vi "Begin.vi"(8 "error in":errorcluster) -> (0 "error out":errorcluster)   [LabVIEW 2019]
doc: "Called before other user functions, this VI can be used to open I/O refnums, load in file data, and do general program initialization. Notice that the <B>error out</B> terminal is simply used for data flow. Wiring it to other structures or subVIs ensures that this VI runs first."
uses:
  <vilib>/Rock Robotics/WPI/DriverStation/WPI_DriverStationRobotMode2.ctl
  <vilib>/Rock Robotics/WPI/Joystick/WPI_JoystickDeviceEnum.ctl
  <vilib>/Rock Robotics/SystemInterfaces/DIO/FPGA_DIOPWMChannel.ctl
  <vilib>/Rock Robotics/WPI/SafetyOutput/WPI_SafetyOutputConfigMenu.ctl
  <vilib>/Rock Robotics/WPI/Solenoid/WPI_SolenoidChannel.ctl
  <vilib>/Rock Robotics/SystemInterfaces/i2clib/i2c_bus.ctl
  <vilib>/Rock Robotics/WPI/Solenoid/WPI_SolenoidValue.ctl
  Robot Global Data.vi
  <vilib>/Rock Robotics/WPI/RobotDrive/WPI_RobotDriveOpen2MotorWithExistingMotors.vi
  <vilib>/Rock Robotics/WPI/MotorControl/WPI_MotorControlOpen SPARK.vi
  <vilib>/Rock Robotics/WPI/Solenoid/WPI_SolenoidOpenDouble.vi
  <vilib>/Rock Robotics/WPI/Solenoid/WPI_SolenoidSetEnum.vi
  <vilib>/Rock Robotics/Network Tables/NT Write Number.vi
  <vilib>/Rock Robotics/Network Tables/NT Write Boolean Array.vi
  <vilib>/Rock Robotics/Network Tables/NT Write Numeric Array.vi
  <vilib>/Rock Robotics/WPI/Ultrasonic/WPI_SonarMB1010DigitalOpen.vi
  <vilib>/Rock Robotics/SystemInterfaces/DIO/FPGA_DIOChannel.ctl
  <vilib>/Rock Robotics/WPI/Ultrasonic/WPI_SonarMB1010DigRefNum Registry Set.vi
panel:
  in  "Blue Calibration":cluster{"R":dbl, "G":dbl, "B":dbl}={"R"=0.143, "G"=0.427, "B"=0.429}
  in  "Green Calibration":cluster{"R":dbl, "G":dbl, "B":dbl}={"R"=0.197, "G"=0.561, "B"=0.24}
  in  "Red Calibration":cluster{"R":dbl, "G":dbl, "B":dbl}={"R"=0.561, "G"=0.323, "B"=0.114}
  in  "Yellow Calibration":cluster{"R":dbl, "G":dbl, "B":dbl}={"R"=0.361, "G"=0.524, "B"=0.113}
  in  "Calibration Time (sec)":u32=4
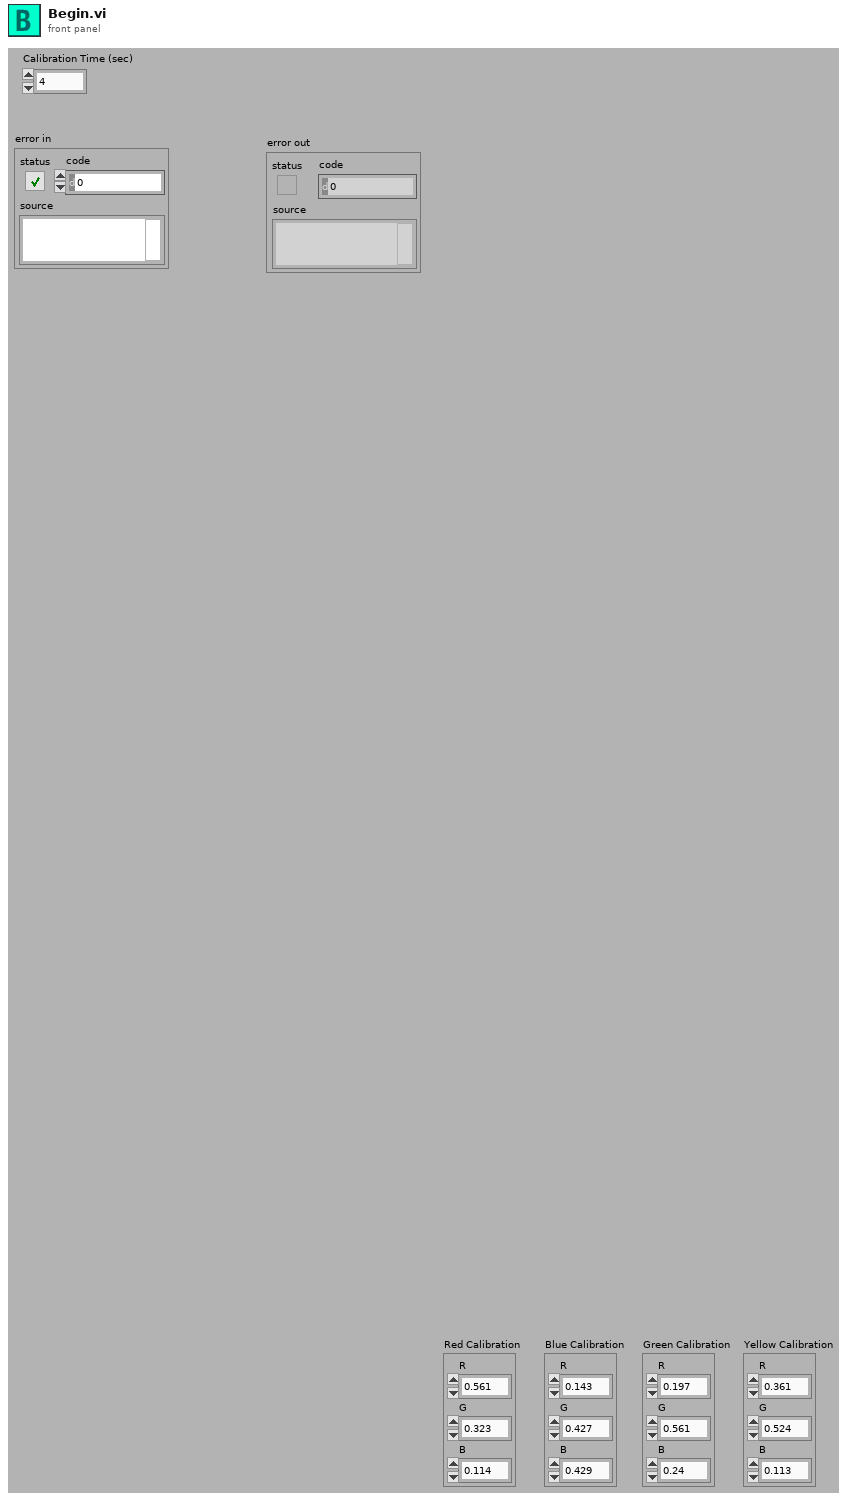
[diagram p1: front panel]
types:
  T1 = typedef "FPGA_DIOChannel.ctl" = enum8{"DIO 0", "DIO 1", "DIO 2", "DIO 3", "DIO 4", "DIO 5", "DIO 6", "DIO 7", "DIO 8", "DIO 9", "DIO MXP 0", "DIO MXP 1", "DIO MXP 2", "DIO MXP 3", "DIO MXP 4", "DIO MXP 5", "DIO MXP 6", "DIO MXP 7", "DIO MXP 8", "DIO MXP 9", "DIO MXP 10", "DIO MXP 11", "DIO MXP 12", "DIO MXP 13", "DIO MXP 14", "DIO MXP 15", "SPI Port CS1", "SPI Port CS2", "SPI Port CS3", "SPI Port MISO", "SPI Port MOSI", "Invalid"}
  T2 = typedef "WPI_SolenoidChannel.ctl" = enum8{"Solenoid 0", "Solenoid 1", "Solenoid 2", "Solenoid 3", "Solenoid 4", "Solenoid 5", "Solenoid 6", "Solenoid 7", "Invalid"}
  T3 = typedef "WPI_SolenoidValue.ctl" = enum16{"Off", "On", "Forward", "Reverse"}
  T4 = typedef "WPI_SafetyOutputConfigMenu.ctl" = enum16{"Enable", "Disable"}
  T5 = typedef "i2c_bus.ctl" = enum16{"I2C On-Board", "I2C MXP", "Invalid"}
  T6 = typedef "FPGA_DIOPWMChannel.ctl" = enum8{"PWM 0", "PWM 1", "PWM 2", "PWM 3", "PWM 4", "PWM 5", "PWM 6", "PWM 7", "PWM 8", "PWM 9", "PWM MXP 0", "PWM MXP 1", "PWM MXP 2", "PWM MXP 3", "PWM MXP 4", "PWM MXP 5", "PWM MXP 6", "PWM MXP 7", "PWM MXP 8", "PWM MXP 9", "Invalid"}
  T7 = typedef "WPI_JoystickDeviceEnum.ctl" = enum16{"USB 0", "USB 1", "USB 2", "USB 3", "USB 4", "USB 5"}
  T8 = typedef "WPI_DriverStationRobotMode2.ctl" = enum16{"Autonomous Disabled", "Autonomous Enabled", "Teleop Disabled", "Teleop Enabled", "Disconnected", "Finish", "Test Disabled", "Test Enabled", "Emergency Stopped"}
  T9 = typedef "WPI_JoystickDevRef.ctl" = cluster{"Device":T7}
  T10 = typedef "WPI_SonarMB1010DigitalDeviceRef.ctl" = cluster{"CounterDevRef":T11, "Scaling factor (s/in)":dbl}
  T11 = typedef "WPI_CounterDevRef.ctl" = cluster{"DevStatus":errorcluster, "CntIndex":T12}
  T12 = typedef "FPGA_CounterCtrSystemIndex.ctl" = enum8{"Ctr 0", "Ctr 1", "Ctr 2", "Ctr 3", "Ctr 4", "Ctr 5", "Ctr 6", "Ctr 7", "Invalid"}
  T13 = typedef "WPI_MotorControlDeviceRef.ctl" = cluster{"DeviceStatus":errorcluster, "Type":T14, "PWM":cluster{"PWM Channel":T6, "DeadBand":T15}, "CAN":cluster{"Device Number":u8, "SetOutput VI Ref":variant, "GetOutput VI Ref":variant, "Enable VI Ref":variant, "Disable VI Ref":variant, "Data":variant}, "Invert":bool, "DIO PWM":cluster{"PWM \"Enable\" Channel":T6, "DIOChannel":T1, "PWM Rate":dbl}}
  T14 = typedef "WPI_MotorControlType.ctl" = enum16{"PWM", "CAN", "DIO PWM"}
  T15 = typedef "WPI_PWMDeadband.ctl" = cluster{"Name":string, "maxPositivePwm":i32, "minPositivePwm":i32, "centerPwm":i32, "maxNegativePwm":i32, "minNegativePwm":i32, "angularRange":u16}
  T16 = typedef "WPI_RobotDriveDevRef.ctl" = cluster{"DevStatus":errorcluster, "Motors[]":T13[], "Square Inputs":bool, "Max Output":dbl}
  T17 = typedef "ADIS 16448 HW Configuration.ctl" = cluster{"SPI Clock Rate (Hz)":dbl, "IMU SPI Mode (3)":T18, "IMU Reset Pin":T1, "IMU SPI Bus":T19, "IMU Data Ready Pin":T1, "Stall Config":cluster{"Pow2BytesPerRead":u8, "StallTicks":u16, "CsToSclkTicks":u8}, "IMU Status LED Pin":T1}
  T18 = typedef "WPI_SPIMode.ctl" = enum16{"Mode 0 (Clk Idle Low,Sample on Leading)", "Mode 1 (Clk Idle Low,Sample on Trailing)", "Mode 2 (Clk Idle High,Sample on Leading)", "Mode 3 (Clk Idle High,Sample on Trailing)"}
  T19 = typedef "spi_bus.ctl" = enum16{"SPI On-Board, CS0", "SPI On-Board, CS1", "SPI On-Board, CS2", "SPI On-Board, CS3", "SPI MXP", "Invalid"}
  T20 = typedef "ADIS16448 Device Reference.ctl" = cluster{"DevStatus":errorcluster, "Hardware Config":T21, "Calibration Complete":refnum<notifier>, "Status FIFO":refnum<k33>, "Last Value Reference":refnum<data-value>, "Sychronous Process VI":T22, "Cmd FIFO":refnum<k33>, "Source":T23, "Data FIFO":refnum<k33>, "IMU Status LED Pin":T1, "Calibration Time":u32}
  T21 = typedef "ADIS16448 Hardware Configuration.ctl" = cluster{"SPI Clock Rate (Hz)":dbl, "IMU SPI Mode (3)":T18, "IMU Reset Pin":T1, "IMU SPI Bus":T19, "IMU Data Ready Pin":T1, "Stall Config":cluster{"Pow2BytesPerRead":u8, "StallTicks":u16, "CsToSclkTicks":u8}, "IMU Status LED Pin":T1}
  T22 = typedef "ADIS16448 Process.ctl" = refnum<vi>
  T23 = typedef "FPGA_CounterEncoderSourceConvertionLVSourceType.ctl" = cluster{"DevStatus":errorcluster, "AnalogTriggerMode?":bool, "DigitalMode":cluster{"DIO Channel":T24}, "AnalogTriggerMode":cluster{"AnalogTriggerIndex":T25, "OutputType":T26}}
  T24 = typedef "FPGA_DIODigitalSourceChannel.ctl" = enum8{"DIO 0", "DIO 1", "DIO 2", "DIO 3", "DIO 4", "DIO 5", "DIO 6", "DIO 7", "DIO 8", "DIO 9", "DIO MXP 0", "DIO MXP 1", "DIO MXP 2", "DIO MXP 3", "DIO MXP 4", "DIO MXP 5", "DIO MXP 6", "DIO MXP 7", "DIO MXP 8", "DIO MXP 9", "DIO MXP 10", "DIO MXP 11", "DIO MXP 12", "DIO MXP 13", "DIO MXP 14", "DIO MXP 15", "SPI Port CS1", "SPI Port CS2", "SPI Port CS3", "SPI Port MISO", "SPI Port MOSI", "Disabled"}
  T25 = typedef "FPGA_AnalogTriggerIndex.ctl" = enum8{"Trig 0", "Trig 1", "Trig 2", "Trig 3", "Trig 4", "Trig 5", "Trig 6", "Trig 7", "Invalid"}
  T26 = typedef "FPGA_AnalogTriggerOutType.ctl" = enum16{"InWindow", "TriggerState", "Rising", "Falling"}
  T27 = typedef "Color Sensor V3 DevRef.ctl" = cluster{"I2CDevRef":T28}
  T28 = typedef "WPI_I2CDevRef.ctl" = cluster{"DevStatus":errorcluster, "Device Address":u8, "Handle":i32, "I2C Bus":T5}
  T29 = typedef "WPI_SolenoidDevRef.ctl" = cluster{"DevStatus":errorcluster, "Pneumatics Control Module":u8, "Forward Solenoid Channel":T2, "Reverse Solenoid Channel":T2}
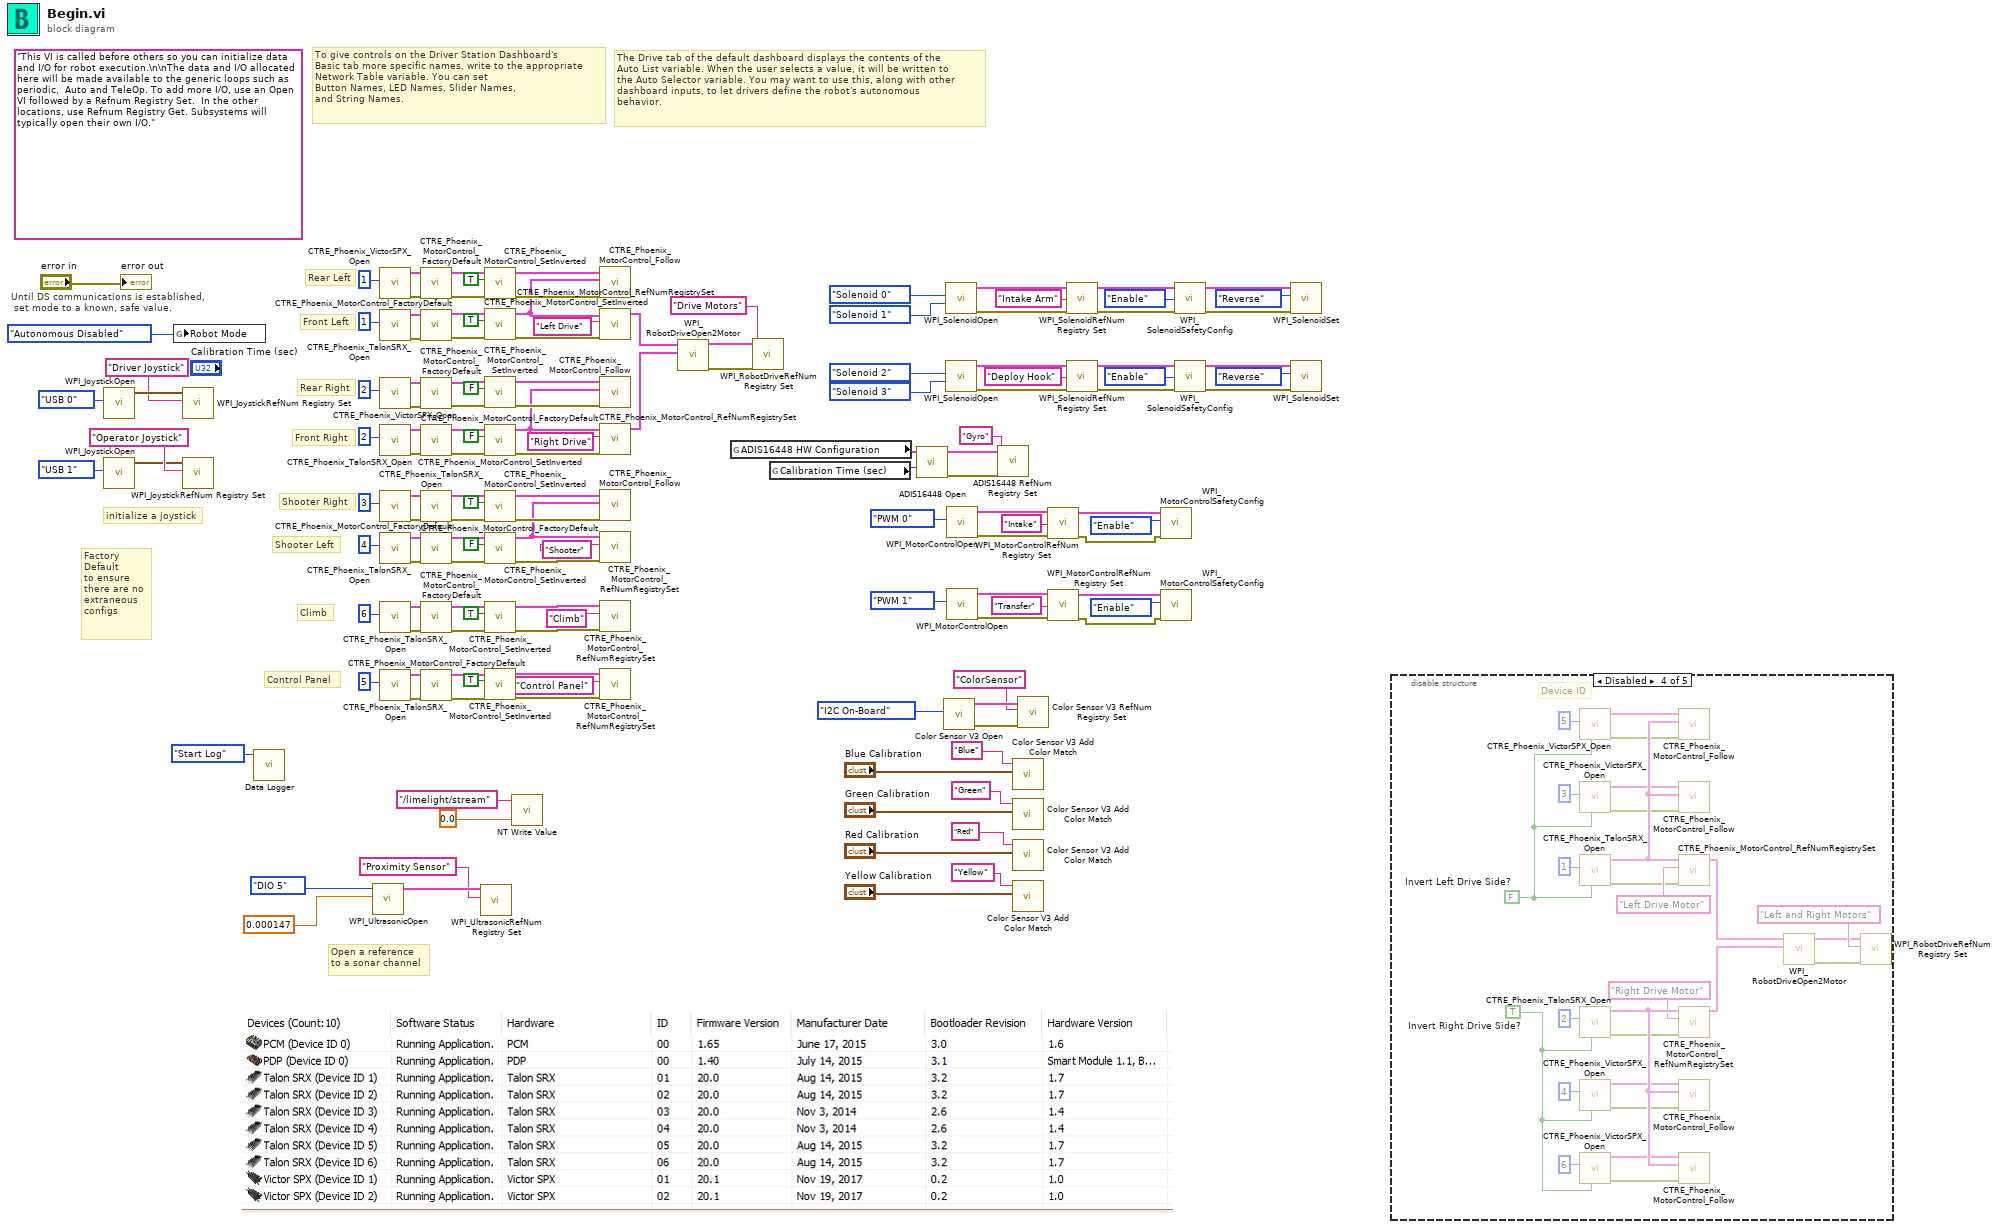
[diagram p0: block diagram]
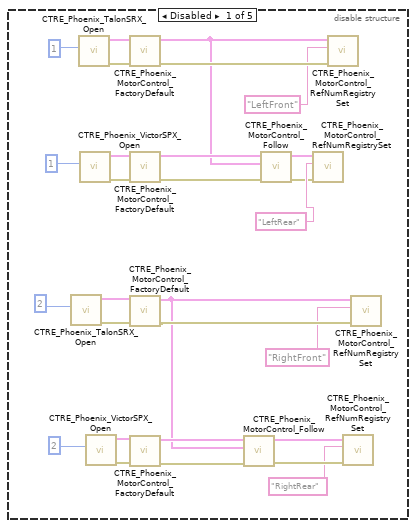
[diagram p2: hidden frame]
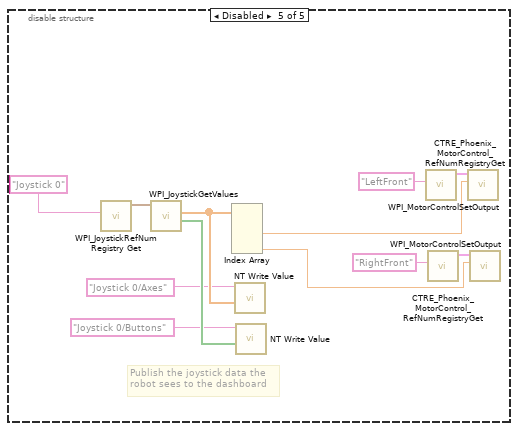
[diagram p5: hidden frame]
diagram:
  (unwired) "This VI is called before others so you can initialize data and I/O for robot execution.\n\nThe data and I/O allocated here will be made available to the generic loops such as periodic,  Auto and TeleOp. To add more I/O, use an Open VI followed by a Refnum Registry Set.  In the other locations, use Refnum Registry Get. Subsystems will typically open their own I/O."
  # "Open a reference\nto a sonar channel"
  # "Climb"
  # "Control Panel"
  # "The Drive tab of the default dashboard displays the contents of the\nAuto List variable. When the user selects a value, it will be written to\nthe Auto Selector variable. You may want to use this, along with other\ndashboard inputs, to let drivers define the robot's autonomous\nbehavior."
  # "To give controls on the Driver Station Dashboard's\nBasic tab more specific names, write to the appropriate\nNetwork Table variable. You can set\nButton Names, LED Names, Slider Names,\nand String Names."
  # "Shooter Left"
  # "Shooter Right"
  # "Factory \nDefault \nto ensure \nthere are no \nextraneous \nconfigs"
  # "Front Right"
  # "Front Left"
  # "Rear Right"
  # "Rear Left"
  # "initialize a joystick"
  # "Until DS communications is established,\n set mode to a known, safe value."
  n1 = call <vilib>:"WPI_JoystickOpen.vi"("JoystickDevice"=WPI_JoystickDeviceEnum."USB 0") -> ("JoystickDevRef"=w125:T9)  [unwired: 10 in]
  n2 = call <vilib>:"WPI_JoystickOpen.vi"("JoystickDevice"=WPI_JoystickDeviceEnum."USB 1") -> ("JoystickDevRef"=w140:T9)  [unwired: 10 in]
  n3 = global write "Robot Global Data.vi" "Robot Mode"(WPI_DriverStationRobotMode2."Autonomous Disabled" ("Robot Mode")) -> ()
  n4 = call <vilib>:"WPI_JoystickRefNum Registry Set.vi"("refnum name"="Driver Joystick", "JoystickDevRef"=w125) -> ()  [unwired: 8 in, 2 out]
  n5 = call <vilib>:"WPI_JoystickRefNum Registry Set.vi"("refnum name"="Operator Joystick", "JoystickDevRef"=w140) -> ()  [unwired: 8 in, 2 out]
  n6 = call "Data Logger.vi"("Function"=enum16{"Start Log", "Log Data", "Stop Log"}."Start Log") -> ()  [unwired: 9 in, 2 out]
  n7 = call-poly <vilib>:"WPI_UltrasonicOpen.vi"("Scaling factor (s/in)"=0.000147, "DIO Channel"=FPGA_DIOChannel."DIO 5") -> ("SonarMB1010DigitalDevRef"=w2:T10)  [unwired: 8 in, 1 out]
  n8 = call <vilib>:"CTRE_Phoenix_VictorSPX_Open.vi"("Device Number"=u8 1) -> ("error out"=w123:errorcluster, "CAN Talon SRX Ref"=w122:T13)  [unwired: 9 in]
  n9 = call <vilib>:"CTRE_Phoenix_TalonSRX_Open.vi"("Device Number"=u8 1) -> ("error out"=w120:errorcluster, "CAN Talon SRX Ref"=w121:T13)  [unwired: 9 in]
  n10 = call <vilib>:"CTRE_Phoenix_VictorSPX_Open.vi"("Device Number"=u8 2) -> ("error out"=w119:errorcluster, "CAN Talon SRX Ref"=w118:T13)  [unwired: 9 in]
  n11 = call <vilib>:"CTRE_Phoenix_TalonSRX_Open.vi"("Device Number"=u8 2) -> ("error out"=w117:errorcluster, "CAN Talon SRX Ref"=w116:T13)  [unwired: 9 in]
  n12 = call <vilib>:"CTRE_Phoenix_TalonSRX_Open.vi"("Device Number"=u8 3) -> ("error out"=w78:errorcluster, "CAN Talon SRX Ref"=w77:T13)  [unwired: 9 in]
  n13 = call <vilib>:"CTRE_Phoenix_TalonSRX_Open.vi"("Device Number"=u8 4) -> ("error out"=w76:errorcluster, "CAN Talon SRX Ref"=w75:T13)  [unwired: 9 in]
  n14 = call <vilib>:"CTRE_Phoenix_TalonSRX_Open.vi"("Device Number"=u8 6) -> ("error out"=w12:errorcluster, "CAN Talon SRX Ref"=w11:T13)  [unwired: 9 in]
  n15 = call <vilib>:"CTRE_Phoenix_TalonSRX_Open.vi"("Device Number"=u8 5) -> ("error out"=w46:errorcluster, "CAN Talon SRX Ref"=w45:T13)  [unwired: 9 in]
  n16 = call <vilib>:"CTRE_Phoenix_MotorControl_FactoryDefault.vi"("error in"=w123, "PhoenixMotorControlDevRef"=w122) -> ("error out"=w114:errorcluster, "PhoenixMotorControlDevRef"=w113:T13)  [unwired: 8 in]
  n17 = call <vilib>:"CTRE_Phoenix_MotorControl_FactoryDefault.vi"("error in"=w120, "PhoenixMotorControlDevRef"=w121) -> ("error out"=w108:errorcluster, "PhoenixMotorControlDevRef"=w109:T13)  [unwired: 8 in]
  n18 = call <vilib>:"CTRE_Phoenix_MotorControl_FactoryDefault.vi"("error in"=w119, "PhoenixMotorControlDevRef"=w118) -> ("error out"=w104:errorcluster, "PhoenixMotorControlDevRef"=w103:T13)  [unwired: 8 in]
  n19 = call <vilib>:"CTRE_Phoenix_MotorControl_FactoryDefault.vi"("error in"=w117, "PhoenixMotorControlDevRef"=w116) -> ("error out"=w99:errorcluster, "PhoenixMotorControlDevRef"=w98:T13)  [unwired: 8 in]
  n20 = call <vilib>:"CTRE_Phoenix_MotorControl_FactoryDefault.vi"("error in"=w78, "PhoenixMotorControlDevRef"=w77) -> ("error out"=w72:errorcluster, "PhoenixMotorControlDevRef"=w73:T13)  [unwired: 8 in]
  n21 = call <vilib>:"CTRE_Phoenix_MotorControl_FactoryDefault.vi"("error in"=w76, "PhoenixMotorControlDevRef"=w75) -> ("error out"=w67:errorcluster, "PhoenixMotorControlDevRef"=w68:T13)  [unwired: 8 in]
  n22 = call <vilib>:"CTRE_Phoenix_MotorControl_FactoryDefault.vi"("error in"=w12, "PhoenixMotorControlDevRef"=w11) -> ("error out"=w8:errorcluster, "PhoenixMotorControlDevRef"=w9:T13)  [unwired: 8 in]
  n23 = call <vilib>:"CTRE_Phoenix_MotorControl_FactoryDefault.vi"("error in"=w46, "PhoenixMotorControlDevRef"=w45) -> ("error out"=w42:errorcluster, "PhoenixMotorControlDevRef"=w43:T13)  [unwired: 8 in]
  n24 = call-poly <vilib>:"WPI_UltrasonicRefNum Registry Set.vi"("refnum name"="Proximity Sensor", "SonarMB1010DigitalDevRef"=w2) -> ()  [unwired: 8 in, 2 out]
  n25 = call <vilib>:"CTRE_Phoenix_MotorControl_SetInverted.vi"("error in (no error)"=w114, "Invert?"=TRUE, "PhoenixMotorControlDevRef"=w113) -> ("error out"=w111:errorcluster, "PhoenixMotorControlDevRef"=w112:T13)  [unwired: 7 in]
  n26 = call <vilib>:"CTRE_Phoenix_MotorControl_SetInverted.vi"("error in (no error)"=w108, "Invert?"=TRUE, "PhoenixMotorControlDevRef"=w109) -> ("error out"=w107:errorcluster, "PhoenixMotorControlDevRef"=w106:T13)  [unwired: 7 in]
  n27 = call <vilib>:"CTRE_Phoenix_MotorControl_SetInverted.vi"("error in (no error)"=w104, "Invert?"=FALSE, "PhoenixMotorControlDevRef"=w103) -> ("error out"=w101:errorcluster, "PhoenixMotorControlDevRef"=w102:T13)  [unwired: 7 in]
  n28 = call <vilib>:"CTRE_Phoenix_MotorControl_SetInverted.vi"("error in (no error)"=w99, "Invert?"=FALSE, "PhoenixMotorControlDevRef"=w98) -> ("error out"=w96:errorcluster, "PhoenixMotorControlDevRef"=w97:T13)  [unwired: 7 in]
  n29 = call <vilib>:"CTRE_Phoenix_MotorControl_SetInverted.vi"("error in (no error)"=w72, "Invert?"=TRUE, "PhoenixMotorControlDevRef"=w73) -> ("error out"=w71:errorcluster, "PhoenixMotorControlDevRef"=w70:T13)  [unwired: 7 in]
  n30 = call <vilib>:"CTRE_Phoenix_MotorControl_SetInverted.vi"("error in (no error)"=w67, "Invert?"=FALSE, "PhoenixMotorControlDevRef"=w68) -> ("error out"=w66:errorcluster, "PhoenixMotorControlDevRef"=w65:T13)  [unwired: 7 in]
  n31 = call <vilib>:"CTRE_Phoenix_MotorControl_SetInverted.vi"("error in (no error)"=w8, "Invert?"=TRUE, "PhoenixMotorControlDevRef"=w9) -> ("error out"=w7:errorcluster, "PhoenixMotorControlDevRef"=w6:T13)  [unwired: 7 in]
  n32 = call <vilib>:"CTRE_Phoenix_MotorControl_SetInverted.vi"("error in (no error)"=w42, "Invert?"=TRUE, "PhoenixMotorControlDevRef"=w43) -> ("error out"=w41:errorcluster, "PhoenixMotorControlDevRef"=w40:T13)  [unwired: 7 in]
  n33 = call-poly <vilib>:"NT Write Value.vi"("Numeric"=0.0, "Name"="/limelight/stream") -> ()  [unwired: 9 in, 1 out]
  n34 = call <vilib>:"CTRE_Phoenix_MotorControl_Follow.vi"("error in (no error)"=w111, "Master Controller to Follow"=w106, "PhoenixMotorControlDevRef"=w112) -> ()  [unwired: 7 in, 2 out]
  n35 = call <vilib>:"CTRE_Phoenix_MotorControl_RefNumRegistrySet.vi"("error in (no error)"=w107, "refnum name"="Left Drive", "PhoenixMotorControlDevRef"=w106) -> ("PhoenixMotorControlDevRef"=w133:T13)  [unwired: 7 in, 1 out]
  n36 = call <vilib>:"CTRE_Phoenix_MotorControl_Follow.vi"("error in (no error)"=w101, "Master Controller to Follow"=w97, "PhoenixMotorControlDevRef"=w102) -> ()  [unwired: 7 in, 2 out]
  n37 = call <vilib>:"CTRE_Phoenix_MotorControl_RefNumRegistrySet.vi"("error in (no error)"=w96, "refnum name"="Right Drive", "PhoenixMotorControlDevRef"=w97) -> ("PhoenixMotorControlDevRef"=w132:T13)  [unwired: 7 in, 1 out]
  n38 = call <vilib>:"CTRE_Phoenix_MotorControl_Follow.vi"("error in (no error)"=w71, "Master Controller to Follow"=w65, "PhoenixMotorControlDevRef"=w70) -> ()  [unwired: 7 in, 2 out]
  n39 = call <vilib>:"CTRE_Phoenix_MotorControl_RefNumRegistrySet.vi"("error in (no error)"=w66, "refnum name"="Shooter", "PhoenixMotorControlDevRef"=w65) -> ()  [unwired: 7 in, 2 out]
  n40 = call <vilib>:"CTRE_Phoenix_MotorControl_RefNumRegistrySet.vi"("error in (no error)"=w7, "refnum name"="Climb", "PhoenixMotorControlDevRef"=w6) -> ()  [unwired: 7 in, 2 out]
  n41 = call <vilib>:"CTRE_Phoenix_MotorControl_RefNumRegistrySet.vi"("error in (no error)"=w41, "refnum name"="Control Panel", "PhoenixMotorControlDevRef"=w40) -> ()  [unwired: 7 in, 2 out]
  n42 = call-poly <vilib>:"WPI_RobotDriveOpen2Motor.vi"("Right Motor Dev Ref"=w132, "Left Motor Dev Ref"=w133) -> ("error out"=w128:errorcluster, "RobotDriveDevRef"=w129:T16)  [unwired: 8 in]
  n43 = global read "Robot Global Data.vi" "ADIS16448 HW Configuration"() -> (w64:T17)
  n44 = call <vilib>:"WPI_RobotDriveRefNum Registry Set.vi"("error in (no error)"=w128, "refnum name"="Drive Motors", "RobotDriveDevRef"=w129) -> ()  [unwired: 7 in, 2 out]
  n45 = global read "Robot Global Data.vi" "Calibration Time (sec)"() -> (w63:u32)
  n46 = call <vilib>:"ADIS16448 Open.vi"("Initial Calibration Time (sec)"=w63, "Hardware Config"=w64) -> ("error out"=w61:errorcluster, "ADIS16448DevRef"=w62:T20)  [unwired: 8 in]
  n47 = call <vilib>:"Color Sensor V3 Open.vi"("I2C Bus"=i2c_bus."I2C On-Board") -> ("error out"=w37:errorcluster, "ColorSensorDevRef"=w38:T27)  [unwired: 9 in]
  n48 = call-poly <vilib>:"WPI_SolenoidOpen.vi"("Reverse Solenoid Channel"=WPI_SolenoidChannel."Solenoid 1" ("Solenoid Channel"), "Forward Solenoid Channel"=WPI_SolenoidChannel."Solenoid 0" ("Solenoid Channel")) -> ("error out"=w56:errorcluster, "SolenoidDevRef"=w59:T29)  [unwired: 8 in]
  n49 = call-poly <vilib>:"WPI_SolenoidOpen.vi"("Reverse Solenoid Channel"=WPI_SolenoidChannel."Solenoid 3" ("Solenoid Channel"), "Forward Solenoid Channel"=WPI_SolenoidChannel."Solenoid 2" ("Solenoid Channel")) -> ("error out"=w19:errorcluster, "SolenoidDevRef"=w16:T29)  [unwired: 8 in]
  n50 = call-poly <vilib>:"WPI_MotorControlOpen.vi"("PWM Channel"=FPGA_DIOPWMChannel."PWM 0") -> ("error out"=w90:errorcluster, "MotorControlDeviceRef"=w94:T13)  [unwired: 9 in]
  n51 = call-poly <vilib>:"WPI_MotorControlOpen.vi"("PWM Channel"=FPGA_DIOPWMChannel."PWM 1") -> ("error out"=w87:errorcluster, "MotorControlDeviceRef"=w83:T13)  [unwired: 9 in]
  n52 = call <vilib>:"ADIS16448 RefNum Registry Set.vi"("error in (no error)"=w61, "refnum name"="Gyro", "ADIS16448DevRef"=w62) -> ()  [unwired: 7 in, 2 out]
  n53 = call <vilib>:"Color Sensor V3 Add Color Match.vi"("Color"="Blue Calibration", "Name"="Blue") -> ()  [unwired: 10 in]
  n54 = call <vilib>:"Color Sensor V3 Add Color Match.vi"("Color"="Green Calibration", "Name"="Green") -> ()  [unwired: 10 in]
  n55 = call <vilib>:"Color Sensor V3 Add Color Match.vi"("Color"="Red Calibration", "Name"="Red") -> ()  [unwired: 10 in]
  n56 = call <vilib>:"Color Sensor V3 Add Color Match.vi"("Color"="Yellow Calibration", "Name"="Yellow") -> ()  [unwired: 10 in]
  n57 = call <vilib>:"Color Sensor V3 RefNum Registry Set.vi"("error in (no error)"=w37, "refnum name"="ColorSensor", "ColorSensorDevRef"=w38) -> ()  [unwired: 7 in, 2 out]
  n58 = call <vilib>:"WPI_MotorControlRefNum Registry Set.vi"("error in (no error)"=w90, "refnum name"="Intake", "MotorControlDevRef"=w94) -> ("error out"=w89:errorcluster, "MotorControlDevRef"=w93:T13)  [unwired: 7 in]
  n59 = call <vilib>:"WPI_MotorControlRefNum Registry Set.vi"("error in (no error)"=w87, "refnum name"="Transfer", "MotorControlDevRef"=w83) -> ("error out"=w88:errorcluster, "MotorControlDevRef"=w84:T13)  [unwired: 7 in]
  n60 = call <vilib>:"WPI_SolenoidRefNum Registry Set.vi"("error in (no error)"=w56, "refnum name"="Intake Arm", "SolenoidDevRef"=w59) -> ("error out"=w55:errorcluster, "SolenoidDevRef"=w58:T29)  [unwired: 7 in]
  n61 = call <vilib>:"WPI_SolenoidRefNum Registry Set.vi"("error in (no error)"=w19, "refnum name"="Deploy Hook", "SolenoidDevRef"=w16) -> ("error out"=w20:errorcluster, "SolenoidDevRef"=w17:T29)  [unwired: 7 in]
  n62 = call <vilib>:"WPI_MotorControlSafetyConfig.vi"("error in (no error)"=w89, "mode"=WPI_SafetyOutputConfigMenu."Enable", "MotorControlDevRef"=w93) -> ()  [unwired: 7 in, 2 out]
  n63 = call <vilib>:"WPI_MotorControlSafetyConfig.vi"("error in (no error)"=w88, "mode"=WPI_SafetyOutputConfigMenu."Enable", "MotorControlDevRef"=w84) -> ()  [unwired: 7 in, 2 out]
  n64 = call <vilib>:"WPI_SolenoidSafetyConfig.vi"("error in (no error)"=w55, "mode"=WPI_SafetyOutputConfigMenu."Enable", "SolenoidDevRef"=w58) -> ("error out"=w54:errorcluster, "SolenoidDevRef"=w57:T29)  [unwired: 7 in]
  n65 = call <vilib>:"WPI_SolenoidSafetyConfig.vi"("error in (no error)"=w20, "mode"=WPI_SafetyOutputConfigMenu."Enable", "SolenoidDevRef"=w17) -> ("error out"=w21:errorcluster, "SolenoidDevRef"=w18:T29)  [unwired: 7 in]
  n66 = call-poly <vilib>:"WPI_SolenoidSet.vi"("error in (no error)"=w54, "Value"=WPI_SolenoidValue."Reverse", "SolenoidDevRef"=w57) -> ()  [unwired: 7 in, 2 out]
  n67 = call-poly <vilib>:"WPI_SolenoidSet.vi"("error in (no error)"=w21, "Value"=WPI_SolenoidValue."Reverse", "SolenoidDevRef"=w18) -> ()  [unwired: 7 in, 2 out]
  n68 = disable-structure shown="Disabled" {
    frame Disabled {
      n69 = call <vilib>:"CTRE_Phoenix_TalonSRX_Open.vi"("Device Number"=u8 2) -> ("error out"=w167:errorcluster, "CAN Talon SRX Ref"=w157:T13)  [unwired: 9 in]
      n70 = call <vilib>:"CTRE_Phoenix_TalonSRX_Open.vi"("Device Number"=u8 1) -> ("error out"=w165:errorcluster, "CAN Talon SRX Ref"=w155:T13)  [unwired: 9 in]
      n71 = call <vilib>:"CTRE_Phoenix_VictorSPX_Open.vi"("Device Number"=u8 1) -> ("error out"=w163:errorcluster, "CAN Talon SRX Ref"=w161:T13)  [unwired: 9 in]
      n72 = call <vilib>:"CTRE_Phoenix_VictorSPX_Open.vi"("Device Number"=u8 2) -> ("error out"=w169:errorcluster, "CAN Talon SRX Ref"=w159:T13)  [unwired: 9 in]
      n73 = call <vilib>:"CTRE_Phoenix_MotorControl_FactoryDefault.vi"("error in"=w165, "PhoenixMotorControlDevRef"=w155) -> ("error out"=w166:errorcluster, "PhoenixMotorControlDevRef"=w156:T13)  [unwired: 8 in]
      n74 = call <vilib>:"CTRE_Phoenix_MotorControl_FactoryDefault.vi"("error in"=w163, "PhoenixMotorControlDevRef"=w161) -> ("error out"=w164:errorcluster, "PhoenixMotorControlDevRef"=w162:T13)  [unwired: 8 in]
      n75 = call <vilib>:"CTRE_Phoenix_MotorControl_FactoryDefault.vi"("error in"=w167, "PhoenixMotorControlDevRef"=w157) -> ("error out"=w168:errorcluster, "PhoenixMotorControlDevRef"=w158:T13)  [unwired: 8 in]
      n76 = call <vilib>:"CTRE_Phoenix_MotorControl_FactoryDefault.vi"("error in"=w169, "PhoenixMotorControlDevRef"=w159) -> ("error out"=w170:errorcluster, "PhoenixMotorControlDevRef"=w160:T13)  [unwired: 8 in]
      n77 = call <vilib>:"CTRE_Phoenix_MotorControl_Follow.vi"("error in (no error)"=w170, "Master Controller to Follow"=w158, "PhoenixMotorControlDevRef"=w160) -> ("error out"=w153:errorcluster, "PhoenixMotorControlDevRef"=w154:T13)  [unwired: 7 in]
      n78 = call <vilib>:"CTRE_Phoenix_MotorControl_Follow.vi"("error in (no error)"=w164, "Master Controller to Follow"=w156, "PhoenixMotorControlDevRef"=w162) -> ("error out"=w145:errorcluster, "PhoenixMotorControlDevRef"=w146:T13)  [unwired: 7 in]
      n79 = call <vilib>:"CTRE_Phoenix_MotorControl_RefNumRegistrySet.vi"("error in (no error)"=w145, "refnum name"="LeftRear", "PhoenixMotorControlDevRef"=w146) -> ()  [unwired: 7 in, 2 out]
      n80 = call <vilib>:"CTRE_Phoenix_MotorControl_RefNumRegistrySet.vi"("error in (no error)"=w166, "refnum name"="LeftFront", "PhoenixMotorControlDevRef"=w156) -> ()  [unwired: 7 in, 2 out]
      n81 = call <vilib>:"CTRE_Phoenix_MotorControl_RefNumRegistrySet.vi"("error in (no error)"=w153, "refnum name"="RightRear", "PhoenixMotorControlDevRef"=w154) -> ()  [unwired: 7 in, 2 out]
      n82 = call <vilib>:"CTRE_Phoenix_MotorControl_RefNumRegistrySet.vi"("error in (no error)"=w168, "refnum name"="RightFront", "PhoenixMotorControlDevRef"=w158) -> ()  [unwired: 7 in, 2 out]
    }
    frame Enabled {
    }
    frame Disabled {
    }
    frame Disabled {
      w197 = FALSE  # Invert Left Drive Side?
      w196 = TRUE  # Invert Right Drive Side?
      # "Device ID"
      n83 = call <vilib>:"CTRE_Phoenix_VictorSPX_Open.vi"("Invert"=w197, "Device Number"=u8 5) -> ("error out"=w187:errorcluster, "CAN Talon SRX Ref"=w188:T13)  [unwired: 8 in]
      n84 = call <vilib>:"CTRE_Phoenix_VictorSPX_Open.vi"("Invert"=w197, "Device Number"=u8 3) -> ("error out"=w186:errorcluster, "CAN Talon SRX Ref"=w189:T13)  [unwired: 8 in]
      n85 = call <vilib>:"CTRE_Phoenix_TalonSRX_Open.vi"("Invert"=w197, "Device Number"=u8 1) -> ("error out"=w177:errorcluster, "CAN Talon SRX Ref"=w190:T13)  [unwired: 8 in]
      n86 = call <vilib>:"CTRE_Phoenix_TalonSRX_Open.vi"("Invert"=w196, "Device Number"=u8 2) -> ("error out"=w178:errorcluster, "CAN Talon SRX Ref"=w185:T13)  [unwired: 8 in]
      n87 = call <vilib>:"CTRE_Phoenix_VictorSPX_Open.vi"("Invert"=w196, "Device Number"=u8 4) -> ("error out"=w181:errorcluster, "CAN Talon SRX Ref"=w182:T13)  [unwired: 8 in]
      n88 = call <vilib>:"CTRE_Phoenix_VictorSPX_Open.vi"("Invert"=w196, "Device Number"=u8 6) -> ("error out"=w184:errorcluster, "CAN Talon SRX Ref"=w183:T13)  [unwired: 8 in]
      n89 = call <vilib>:"CTRE_Phoenix_MotorControl_Follow.vi"("error in (no error)"=w187, "Master Controller to Follow"=w190, "PhoenixMotorControlDevRef"=w188) -> ()  [unwired: 7 in, 2 out]
      n90 = call <vilib>:"CTRE_Phoenix_MotorControl_Follow.vi"("error in (no error)"=w186, "Master Controller to Follow"=w190, "PhoenixMotorControlDevRef"=w189) -> ()  [unwired: 7 in, 2 out]
      n91 = call <vilib>:"CTRE_Phoenix_MotorControl_RefNumRegistrySet.vi"("error in (no error)"=w177, "refnum name"="Left Drive Motor", "PhoenixMotorControlDevRef"=w190) -> ("PhoenixMotorControlDevRef"=w191:T13)  [unwired: 7 in, 1 out]
      n92 = call <vilib>:"CTRE_Phoenix_MotorControl_RefNumRegistrySet.vi"("error in (no error)"=w178, "refnum name"="Right Drive Motor", "PhoenixMotorControlDevRef"=w185) -> ("PhoenixMotorControlDevRef"=w192:T13)  [unwired: 7 in, 1 out]
      n93 = call <vilib>:"CTRE_Phoenix_MotorControl_Follow.vi"("error in (no error)"=w181, "Master Controller to Follow"=w185, "PhoenixMotorControlDevRef"=w182) -> ()  [unwired: 7 in, 2 out]
      n94 = call <vilib>:"CTRE_Phoenix_MotorControl_Follow.vi"("error in (no error)"=w184, "Master Controller to Follow"=w185, "PhoenixMotorControlDevRef"=w183) -> ()  [unwired: 7 in, 2 out]
      n95 = call-poly <vilib>:"WPI_RobotDriveOpen2Motor.vi"("Right Motor Dev Ref"=w192, "Left Motor Dev Ref"=w191) -> ("error out"=w193:errorcluster, "RobotDriveDevRef"=w194:T16)  [unwired: 8 in]
      n96 = call <vilib>:"WPI_RobotDriveRefNum Registry Set.vi"("error in (no error)"=w193, "refnum name"="Left and Right Motors", "RobotDriveDevRef"=w194) -> ()  [unwired: 7 in, 2 out]
    }
    frame Disabled {
      # "Publish the joystick data the\nrobot sees to the dashboard"
      n97 = call <vilib>:"WPI_JoystickRefNum Registry Get.vi"("refnum name"="Joystick 0") -> ("JoystickDevRef"=w199:T9)  [unwired: 1 in, 9 out]
      n98 = call <vilib>:"WPI_JoystickGetValues.vi"("JoystickDevRef"=w199) -> ("Buttons"=w203:bool[], "Axes"=w202:dbl[])  [unwired: 6 in, 3 out]
      n99 = Index Array(array=w202) -> (element #2=w206:dbl, element #4=w209:dbl)  [unwired: 4 in, 2 out]
      n100 = call-poly <vilib>:"NT Write Value.vi"("Numeric Array"=w202, "Name"="Joystick 0/Axes") -> ()  [unwired: 9 in, 1 out]
      n101 = call-poly <vilib>:"NT Write Value.vi"("Boolean Array"=w203, "Name"="Joystick 0/Buttons") -> ()  [unwired: 9 in, 1 out]
      n102 = call <vilib>:"CTRE_Phoenix_MotorControl_RefNumRegistryGet.vi"("refnum name"="LeftFront") -> ("PhoenixMotorControlDevRef"=w205:T13)  [unwired: 9 in, 1 out]
      n103 = call <vilib>:"CTRE_Phoenix_MotorControl_RefNumRegistryGet.vi"("refnum name"="RightFront") -> ("PhoenixMotorControlDevRef"=w208:T13)  [unwired: 9 in, 1 out]
      n104 = call <vilib>:"WPI_MotorControlSetOutput.vi"("Output"=w206, "MotorControlDevRef"=w205) -> ()  [unwired: 7 in, 3 out]
      n105 = call <vilib>:"WPI_MotorControlSetOutput.vi"("Output"=w209, "MotorControlDevRef"=w208) -> ()  [unwired: 7 in, 3 out]
    }
  }
  "error out" <- "error in"
